vi "UDP ESSENTIAL SENDER.vi"(7 "milliseconds to wait (LoopTimer)":u32, 8 "error in (no error)":errorcluster, 9 "destination adress":string, 10 "destination port":u16, 11 "UDP Network Connection in":refnum<k16>) -> (0 "error out":errorcluster)   [LabVIEW 2016]
uses:
  Globale Variablen VI/AutonomousMode.vi
  Globale Variablen VI/Global Variables.vi
  Globale Variablen VI/RadSensoren.vi
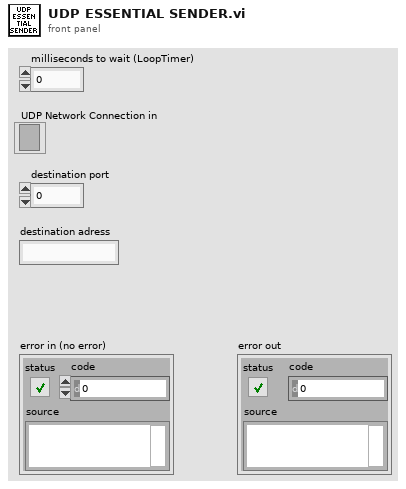
[diagram p1: front panel]
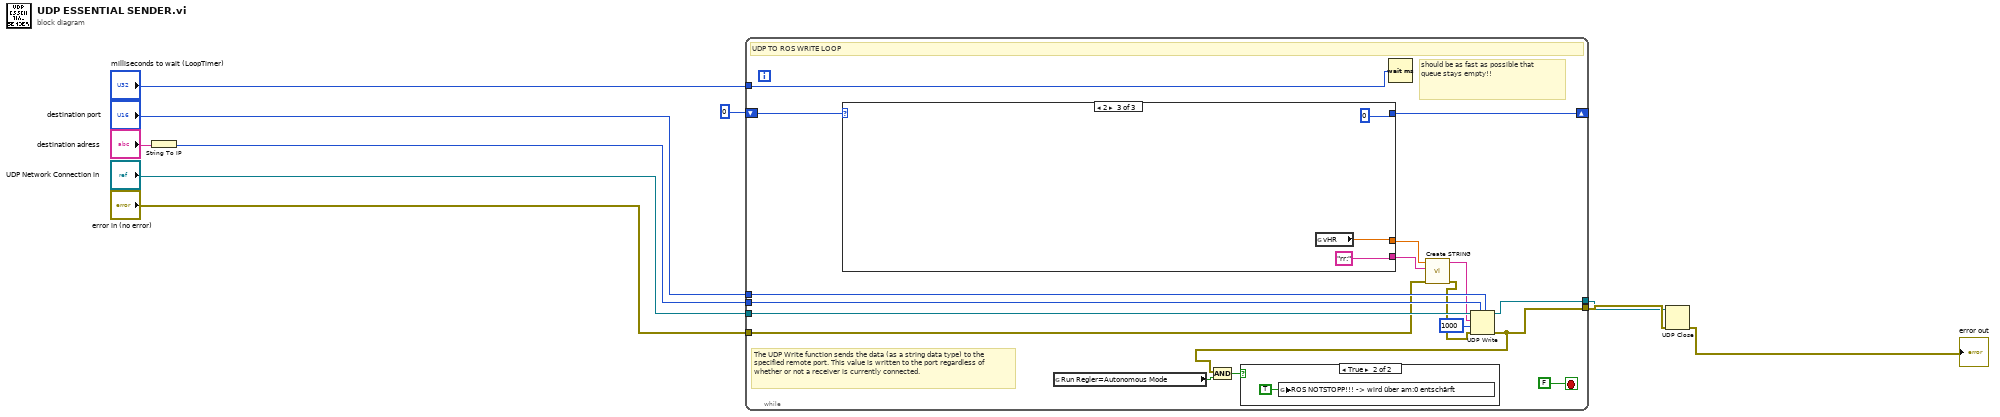
[diagram p0: block diagram]
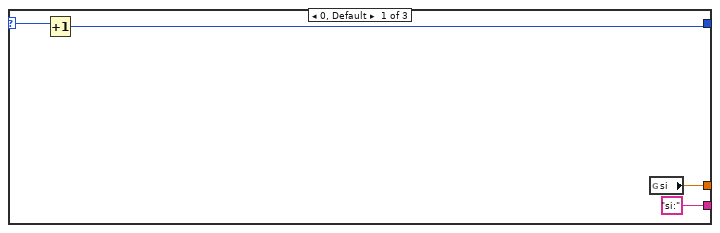
[diagram p3: hidden frame]
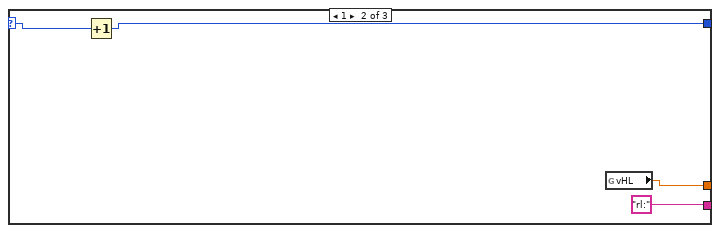
[diagram p4: hidden frame]
diagram:
  n1 = String To IP(1:"destination adress") -> (0:w7:u32)
  n2 = while {
    tunnel: [w12] -> w9
    tunnel: "destination port" -> [w27]
    tunnel: w7 -> [w26]
    tunnel: "UDP Network Connection in" -> [w25]
    tunnel: "error in (no error)" -> [w17]
    tunnel: [w24] -> w8
    tunnel: "milliseconds to wait (LoopTimer)" -> [w23]
    shift-right: [w21] -> _
    shift-left: 0 -> [w20]
    stop <- FALSE stop-if-true
    # "should be as fast as possible that queue stays empty!!"
    # "The UDP Write function sends the data (as a string data type) to the specified remote port. This value is written to the port regardless of whether or not a receiver is currently connected."
    # "UDP TO ROS WRITE LOOP"
    n3 = case shown="2" w20 {
      selector: w20 -> [w30 w34 _]
      tunnel: [w29 w33 0] -> w21
      tunnel: [w32 w36 w39] -> w19
      tunnel: ["si:" "rl:" "rr:"] -> w18
      frame 0, Default {
        n4 = Increment(x=w30) -> (x+1=w29:i32)
        n5 = global read "Global Variables.vi" "si"() -> (w32:dbl)
      }
      frame 1 {
        n6 = Increment(x=w34) -> (x+1=w33:i32)
        n7 = global read "RadSensoren.vi" "vHL"() -> (w36:sgl)
      }
      frame 2 {
        n8 = global read "RadSensoren.vi" "vHR"() -> (w39:sgl)
      }
    }
    n9 = global read "AutonomousMode.vi" "Run Regler=Autonomous Mode"() -> (w13:bool)
    n10 = Wait (ms)(milliseconds to wait=w23) -> ()  [unwired: 1 out]
    n11 = call "Create STRING.vi"("error in (no error)"=w17, "Descriptor"=w18, "Value IN"=w19) -> ("error out"=w16:errorcluster, "concatenated string"=w15:string)  [unwired: 7 in]
    n12 = UDP Write(address=w26, port or service name=w27, connection ID=w25, data in=w15, 8:w16, 9:1000 ("timeout ms (25000)")) -> (error out=w12:errorcluster, 3:w24:refnum<k16>)
    n13 = And(x=w12, y=w13) -> (x .and. y?=w14:bool)
    n14 = case shown="True" w14 {
      frame False {
      }
      frame True {
        n15 = global write "AutonomousMode.vi" "ROS NOTSTOPP!!! -> wird über am:0 entschärft"(TRUE ("ROS NOTSTOPP!!! -> wird über am:0 entschärft")) -> ()
      }
    }
  }
  n16 = UDP Close(connection ID=w8, 8:w9) -> (error out=→"error out":errorcluster)  [unwired: 1 out]
